vi "BRig_generic_convert__Prob_to_TrueFalse__boolean.vi"(11 "input_probability_u16":u16) -> (3 "output_TF":bool)   [LabVIEW 2014]
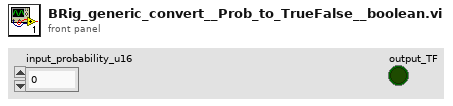
[diagram p1: front panel]
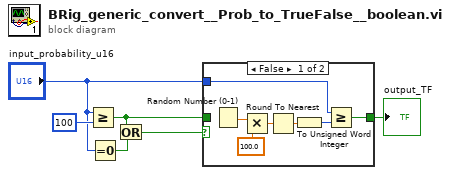
[diagram p0: block diagram]
diagram:
  n1 = Greater Or Equal?(x="input_probability_u16", y=u16 100) -> (x >= y?=w3:bool)
  n2 = Equal To 0?(x="input_probability_u16") -> (x = 0?=w5:bool)
  n3 = Or(x=w3, y=w5) -> (x .or. y?=w4:bool)
  n4 = case shown="False" w4 {
    tunnel: w3 -> [_ w14]
    tunnel: [w7 w14] -> w2
    tunnel: "input_probability_u16" -> [w8 _]
    frame False {
      n5 = Random Number (0-1)() -> (number: 0 to 1=w9:dbl)
      n6 = Multiply(x=w9, y=100.0) -> (x*y=w10:dbl)
      n7 = Round To Nearest(number=w10) -> (nearest integer value=w11:dbl)
      n8 = To Unsigned Word Integer(number=w11) -> (unsigned 16bit integer=w12:u16)
      n9 = Greater Or Equal?(x=w8, y=w12) -> (x >= y?=w7:bool)
    }
    frame True {
    }
  }
  "output_TF" <- w2
